vi "串口通讯实验.vi"() -> ()   [LabVIEW 2018]
uses:
  D:/Program Files (x86)/National Instruments/LabVIEW 2018/examples/Instrument IO/Serial/support/Serial - Settings.ctl
  D:/Program Files (x86)/National Instruments/LabVIEW 2018/examples/Instrument IO/Serial/support/Serial - XON-XOFF Characters.ctl
  D:/Program Files (x86)/National Instruments/LabVIEW 2018/examples/Instrument IO/Serial/support/Serial - ASCII Characters.ctl
  <vilib>/Instr/_visa.llb/VISA Configure Serial Port (Instr).vi
panel:
  out "读取次数":dbl
  in  "终止符":u8=10 format="%.0x"
  in  "终止符时结束写入？":bool=TRUE
  in  "VISA资源名称":refnum<visa-resource-name>="COM1"
  in  "XON/XOFF字符":T1={"XON"=enum."DC1", "XOFF"=enum."DC3"}
  in  "串口设置":T3={"波特率"=9600, "数据位"=8, "校验"=enum."None", "停止位"=10, "流控制"=0} {"流控制" items=["无"=0, "XON/XOFF"=1, "RTS/CTS"=2, "DTR/DSR"=4]; "停止位" items=["1.0"=10, "1.5"=15, "2.0"=20]; "数据位" min=5 max=8 step=1; "波特率" items=["75"=75, "110"=110, "134"=134, "150"=150, "300"=300, "600"=600, "1200"=1200, "1800"=1800, "2400"=2400, "4800"=4800, "7200"=7200, "9600"=9600, "14400"=14400, "19200"=19200, "28800"=28800, "38400"=38400, "56000"=56000, "57600"=57600, "115200"=115200, "128000"=128000, "230400"=230400]}
  in  "终止符时结束读取？":bool=TRUE
  out "响应":string
  in  "读数":u32=1000
  in  "命令":string="*IDN?"
  in  "读取":bool
  in  "停止":bool
  in  "写入":bool
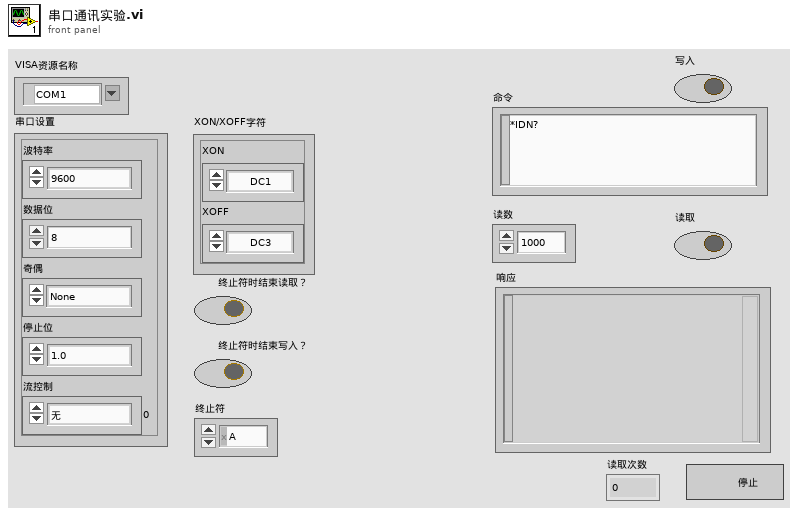
[diagram p1: front panel]
types:
  T1 = typedef "Serial - XON-XOFF Characters.ctl" = cluster{"XON":T2, "XOFF":T2}
  T2 = typedef "Serial - ASCII Characters.ctl" = enum16{"NUL", "SOH", "STX", "ETX", "EOT", "ENQ", "ACK", "BEL", "BS", "HT", "LF", "VT", "FF", "CR", "SO", "SI", "DLE", "DC1", "DC2", "DC3", "DC4", "NAK", "SYN", "ETB", "CAN", "EM", "SUB", "ESC", "FS", "GS", "RS", "US", "SP", "!", "\"", "#", "$", "%", "&", "'", "(", ")", "*", "+", ",", "- (-)", ".", "/", "0", "1", "2", "3", "4", "5", "6", "7", "8", "9", ":", ";", "<", "=", ">", "?", "@", "A", "B", "C", "D", "E", "F", "G", "H", "I", "J", "K", "L", "M", "N", "O", "P", "Q", "R", "S", "T", "U", "V", "W", "X", "Y", "Z", "[", "\\", "]", "^", "_", "`", "a", "b", "c", "d", "e", "f", "g", "h", "i", "j", "k", "l", "m", "n", "o", "p", "q", "r", "s", "t", "u", "v", "w", "x", "y", "z", "{", "|", "}", "~"}
  T3 = typedef "Serial - Settings.ctl" = cluster{"波特率":u32, "数据位":u16, "校验":enum16{"None", "Odd", "Even", "Mark", "Space"}, "停止位":u16, "流控制":u16}
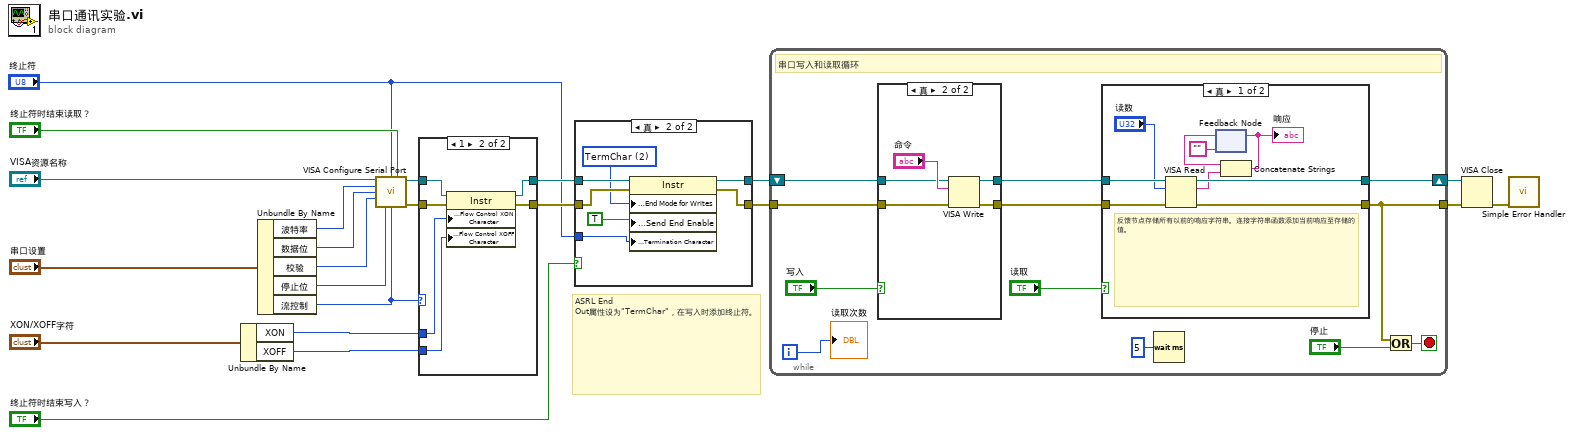
[diagram p0: block diagram]
diagram:
  # "ASRL End Out属性设为\"TermChar\"，在写入时添加终止符。"
  n1 = Unbundle By Name("XON/XOFF字符") -> ("XON"=w8:T2, "XOFF"=w7:T2)
  n2 = Unbundle By Name("串口设置") -> ("波特率"=w15:u32, "数据位"=w16:u16, "校验"=w17:enum16{"None", "Odd", "Even", "Mark", "Space"}, "停止位"=w18:u16, "流控制"=w9:u16)
  n3 = call-poly "VISA Configure Serial Port"("VISA resource name"="VISA资源名称", "termination char\n(0xA = '\\n' = LF)"="终止符", "Enable Termination\nChar (T)"="终止符时结束读取？", "baud rate (9600)"=w15, "data bits (8)"=w16, "parity (0:none)"=w17, "stop bits (10: 1 bit)"=w18, "flow control (0:none)"=w9) -> ("VISA resource name out"=w19:refnum<visa-resource-name>, "error out"=w20:errorcluster)  [unwired: 2 in, 4 out]
  n4 = case shown="1" w9 {
    tunnel: [w23 w30] -> w6
    tunnel: [w24 w29] -> w4
    tunnel: w20 -> [w23 w28]
    tunnel: w19 -> [w24 w27]
    tunnel: w8 -> [_ w26]
    tunnel: w7 -> [_ w25]
    frame Default {
    }
    frame 1 {
      n5 = property on="属性节点" class="Instr"(reference=w27, error in=w28, "Serial Settings:Flow Control XON Character"=w26, "Serial Settings:Flow Control XOFF Character"=w25) -> (reference out=w29:refnum<visa-resource-name>, error out=w30:errorcluster)
    }
  }
  n6 = case shown="真" "终止符时结束写入？" {
    tunnel: w4 -> [w31 w39]
    tunnel: w6 -> [w32 w38]
    tunnel: [w31 w37] -> w3
    tunnel: [w32 w36] -> w5
    tunnel: "终止符" -> [_ w34]
    frame False {
    }
    frame True {
      w35 = u16 2 items=["None", "LastBit", "TermChar", "Break"] ("Serial Settings:Serial End Mode for Writes")
      n7 = property class="Instr"(reference=w39, error in=w38, "Serial Settings:End Mode for Writes"=w35, "Message Based Settings:Send End Enable"=TRUE, "Message Based Settings:Termination Character"=w34) -> (reference out=w37:refnum<visa-resource-name>, error out=w36:errorcluster)
    }
  }
  n8 = while {
    shift-right: [w51] -> w10
    shift-left: w3 -> [w50]
    tunnel: w5 -> [w49]
    tunnel: [w43] -> w11
    i -> [w40]
    stop <- w44 stop-if-true
    # "串口写入和读取循环"
    n9 = case shown="真" "写入" {
      tunnel: w50 -> [w53 w57]
      tunnel: w49 -> [w52 w56]
      tunnel: [w53 w55] -> w48
      tunnel: [w52 w54] -> w47
      frame False {
      }
      frame True {
        n10 = VISA Write(VISA resource name=w57, write buffer="命令", error in (no error)=w56) -> (VISA resource name out=w55:refnum<visa-resource-name>, error out=w54:errorcluster)  [unwired: 1 out]
      }
    }
    n11 = case shown="真" "读取" {
      tunnel: [w65 w69] -> w51
      tunnel: w48 -> [w67 w69]
      tunnel: [w63 w68] -> w43
      tunnel: w47 -> [w66 w68]
      frame True {
        # "反馈节点存储所有以前的响应字符串。连接字符串函数添加当前响应至存储的值。"
        n12 = VISA Read(VISA resource name=w67, byte count="读数", error in (no error)=w66) -> (VISA resource name out=w65:refnum<visa-resource-name>, read buffer=w62:string, error out=w63:errorcluster)  [unwired: 1 out]
        n13 = feedback #1("") -> (w61:string)
        n14 = Concatenate Strings(w61, w62) -> (w60:string)
        "响应" <- w60
        n15 = feedback-in #1(w60) -> ()
      }
      frame False {
      }
    }
    n16 = Wait (ms)(milliseconds to wait=u32 5) -> ()  [unwired: 1 out]
    n17 = Or(x=w43, y="停止") -> (x .or. y?=w44:bool)
    "读取次数" <- w40
  }
  n18 = VISA Close(VISA resource name=w10, error in (no error)=w11) -> (error out=w12:errorcluster)
  n19 = call <vilib>:"Simple Error Handler.vi"("error in (no error)"=w12) -> ()  [unwired: 1 in, 8 out]
